vi "Polling.vi"(8 "Error In":errorcluster, 11 "CS++BaseActor in":refnum<class "CS++BaseActor.lvclass">) -> (0 "Error Out":errorcluster, 3 "CS++BaseActor out":refnum<class "CS++BaseActor.lvclass">)   [LabVIEW 2016, in "CS++BaseActor.lvlib" / "CS++BaseActor.lvclass"]
doc: "This public static VI calls the Polling Core.vi, which can be overritten by a derived class, and publishes the polling time."
uses:
  CS++BaseActor.lvclass
  C:/Program Files (x86)/National Instruments/LabVIEW 2016/vi.lib/ActorFramework/Actor/Actor.lvclass
  CS++BaseActor.lvclass/CS++BaseActor.ctl
  <vilib>/ActorFramework/Actor/Actor.lvclass/Actor.ctl
  <vilib>/ActorFramework/Message Enqueuer/Message Enqueuer.lvclass/Message Enqueuer.ctl
  Libraries/Base/Severity.ctl
  Classes/CS++ProcessVariables/ProcessVariable/PV.lvclass
  Classes/CS++ProcessVariables/ProcessVariable/PV.lvclass/PV.ctl
  Classes/CS++ProcessVariables/ProcessVariable/Write Data.vi
  Classes/CS++ProcessVariables/ProcessVariable/Write Timestamp.vi
  <vilib>/ActorFramework/Message Enqueuer/Init from Existing Queue.vi
  <vilib>/ActorFramework/Message Enqueuer/Enqueue.vi
  CS++BaseActor Messages/Polling Msg/Polling Msg.lvclass
  C:/Program Files (x86)/National Instruments/LabVIEW 2016/vi.lib/ActorFramework/Message/Message.lvclass
  <vilib>/ActorFramework/Message Priority Queue/Priority Enqueue.vi
  <vilib>/ActorFramework/Message Enqueuer/Message Enqueuer.lvclass
  <vilib>/ActorFramework/Actor/Actor.lvclass
  Libraries/Utilities/CS++Utilities.lvlib
  Libraries/Base/CS++Base.lvlib
  Classes/CS++ProcessVariables/PVConnection/PVConnection.lvclass
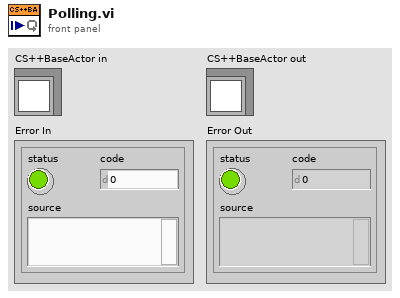
[diagram p1: front panel]
types:
  T1 = typedef "CS++Base.lvlib/Severity.ctl" = enum16{"emergency", "alert", "critical", "error", "warning", "notice", "info", "debug"}
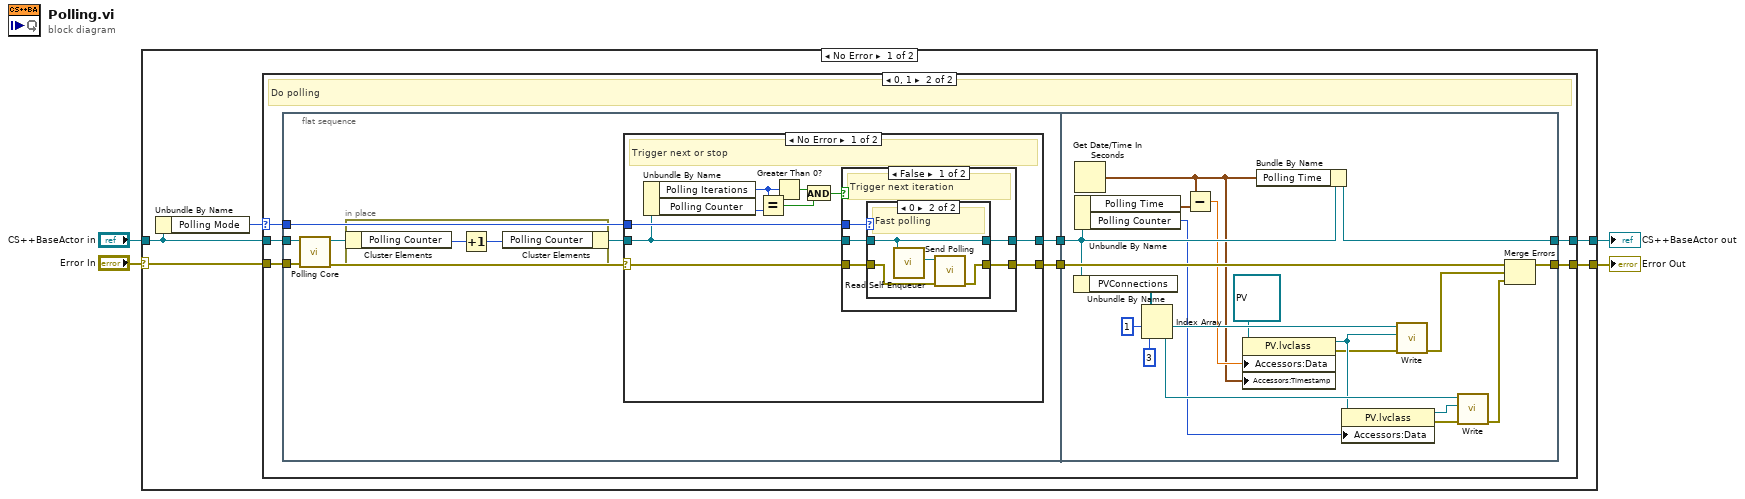
[diagram p0: block diagram]
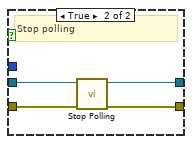
[diagram p4: hidden frame]
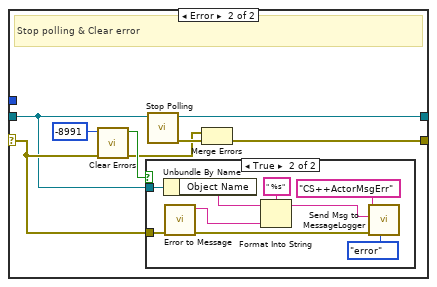
[diagram p5: hidden frame]
diagram:
  n1 = case shown="No Error" "Error In" {
    selector: "Error In" -> [w9 w92]
    tunnel: [w8 w92] -> w3
    tunnel: [w7 w91] -> w1
    tunnel: "CS++BaseActor in" -> [w6 w91]
    frame No Error {
      n2 = Unbundle By Name(w6) -> ("Polling Mode"=w5:i32)
      n3 = case shown="0, 1" w5 {
        selector: w5 -> [_ w14]
        tunnel: w9 -> [w10 w18]
        tunnel: [w10 w17] -> w8
        tunnel: [w11 w16] -> w7
        tunnel: w6 -> [w11 w15]
        frame -1, Default {
          # "Do nothing"
        }
        frame 0, 1 {
          # "Do polling"
          n4 = flat-sequence {
            tunnel: w18 -> [w26]
            tunnel: w15 -> [w23]
            tunnel: w14 -> [w21]
            tunnel: [w25] -> w13
            tunnel: [w24] -> w12
            tunnel: [w90] -> w16
            tunnel: [w81] -> w17
            tunnel: w13 -> [w88]
            tunnel: w12 -> [w87]
            frame #0 {
              n5 = call-dynamic "Polling Core.vi"("Error In"=w26, "CS++BaseActor in"=w23) -> ("Error Out"=w22:errorcluster, "CS++BaseActor out"=w20:refnum<class "CS++BaseActor.lvclass">)  [unwired: 8 in]
              n6 = in-place {
                n7 = in-place-cluster #1(w20) -> ("Polling Counter"=w28:u32)
                n8 = Increment(x=w28) -> (x+1=w27:u32)
                n9 = in-place-cluster #1("Polling Counter"=w27) -> (w19:refnum<class "CS++BaseActor.lvclass">)
              }
              n10 = case shown="No Error" w22 {
                selector: w22 -> [w38 w57]
                tunnel: w19 -> [w34 w54]
                tunnel: [w35 w60] -> w24
                tunnel: [w37 w56] -> w25
                tunnel: w21 -> [w36 _]
                frame No Error {
                  # "Trigger next or stop"
                  n11 = Unbundle By Name(w34) -> ("Polling Iterations"=w32:u32, "Polling Counter"=w33:u32)
                  n12 = Equal?(x=w32, y=w33) -> (x = y?=w30:bool)
                  n13 = Greater Than 0?(x=w32) -> (x > 0?=w31:bool)
                  n14 = And(x=w31, y=w30) -> (x .and. y?=w29:bool)
                  n15 = case shown="False" w29 {
                    tunnel: w38 -> [w43 w52]
                    tunnel: [w42 w51] -> w37
                    tunnel: w36 -> [w41 _]
                    tunnel: [w40 w50] -> w35
                    tunnel: w34 -> [w39 w53]
                    frame False {
                      # "Trigger next iteration"
                      n16 = case shown="0" w41 {
                        tunnel: w39 -> [w45 w46]
                        tunnel: w43 -> [w44 w49]
                        tunnel: [w44 w48] -> w42
                        tunnel: [w45 w46] -> w40
                        frame -1, 1, Default {
                          # "Do nothing"
                        }
                        frame 0 {
                          # "Fast polling"
                          n17 = call <vilib>:"Read Self Enqueuer.vi"("Actor"=w46) -> ("Self Enqueuer"=w47:refnum<class "Message Enqueuer.lvclass">)  [unwired: 10 in]
                          n18 = call "Send Polling.vi"("error in (no error)"=w49, "Message Enqueuer"=w47) -> ("error out"=w48:errorcluster)  [unwired: 8 in, 1 out]
                        }
                      }
                    }
                    frame True {
                      # "Stop polling"
                      n19 = call "Stop Polling.vi"("Error In"=w52, "CS++BaseActor in"=w53) -> ("Error Out"=w51:errorcluster, "CS++BaseActor out"=w50:refnum<class "CS++BaseActor.lvclass">)  [unwired: 8 in]
                    }
                  }
                }
                frame Error {
                  # "Stop polling & Clear error"
                  n20 = call <vilib>:"Clear Errors.vi"("error in (no error)"=w57, "specific error code to clear (0: all)"=-8991 ("Error Code (0)")) -> ("error out"=w55:errorcluster, "specific error cleared?"=w58:bool)  [unwired: 4 in]
                  n21 = case shown="True" w58 {
                    tunnel: w57 -> [_ w68]
                    tunnel: w54 -> [_ w69]
                    frame False {
                    }
                    frame True {
                      n22 = Unbundle By Name(w69) -> ("Object Name"=w65:string)
                      n23 = call "Error to Message.vi"("Error In"=w68) -> ("Error Out"=w67:errorcluster, "Error Message"=w64:string)  [unwired: 9 in]
                      n24 = Format Into String(format string=" %s", initial string=w65, w64) -> (resulting string=w62:string)  [unwired: 1 in, 1 out]
                      n25 = call "Send Msg to MessageLogger.vi"("Severity Code (info)"=Severity."error", "Error In"=w67, "Message Content"=w62, "Message Tag"="CS++ActorMsgErr") -> ()  [unwired: 7 in, 1 out]
                    }
                  }
                  n26 = call "Stop Polling.vi"("CS++BaseActor in"=w54) -> ("Error Out"=w59:errorcluster, "CS++BaseActor out"=w60:refnum<class "CS++BaseActor.lvclass">)  [unwired: 9 in]
                  n27 = Merge Errors(w55, w59) -> (w56:errorcluster)
                }
              }
            }
            frame #1 {
              n28 = Unbundle By Name(w87) -> ("PVConnections"=w86:refnum<class "PVConnection.lvclass">[])
              n29 = Get Date/Time In Seconds() -> (seconds since 1Jan1904=w82:timestamp)
              n30 = Unbundle By Name(w87) -> ("Polling Time"=w89:timestamp, "Polling Counter"=w74:u32)
              n31 = Index Array(array=w86, index #1=1 ("index"), index #2=3 ("index")) -> (element #1=w85:refnum<class "PVConnection.lvclass">, element #2=w77:refnum<class "PVConnection.lvclass">)
              n32 = Subtract(x=w82, y=w89) -> (x-y=w83:dbl)
              n33 = property class="PV.lvclass"(reference=refnum<class "PV.lvclass"> refnum ("CS++ProcessVariables.lvlib:PV.lvclass"), "Accessors:Data"=w83, "Accessors:Timestamp"=w82) -> (reference out=w76:refnum<class "PV.lvclass">, error out=w71:errorcluster)  [unwired: 1 in]
              n34 = Bundle By Name(cluster=w87, "Polling Time"=w82) -> (w90:refnum<class "CS++BaseActor.lvclass">)
              n35 = property class="PV.lvclass"(reference=w76, "Accessors:Data"=w74) -> (reference out=w75:refnum<class "PV.lvclass">, error out=w72:errorcluster)  [unwired: 1 in]
              n36 = call "Write.vi"("error in (no error)"=w71, "PV"=w76, "PVConnection in"=w85) -> ("error out"=w80:errorcluster)  [unwired: 7 in, 1 out]
              n37 = call "Write.vi"("error in (no error)"=w72, "PV"=w75, "PVConnection in"=w77) -> ("error out"=w73:errorcluster)  [unwired: 7 in, 1 out]
              n38 = Merge Errors(w88, w80, w73) -> (w81:errorcluster)
            }
          }
        }
      }
    }
    frame Error {
    }
  }
  "Error Out" <- w3
  "CS++BaseActor out" <- w1
